vi "Close Private Data Cluster Refs.vi"(8 "error in (no error)":errorcluster, 11 "Private Data Refs":T1) -> (0 "error out":errorcluster)   [LabVIEW 2020, in "Add to Private Data.lvlib"]
uses:
  Add to Private Data.lvlib
  Private Data Refs.ctl
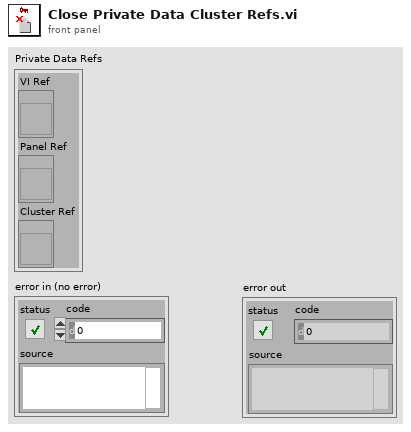
[diagram p1: front panel]
types:
  T1 = typedef "Add to Private Data.lvlib/Private Data Refs.ctl" = cluster{"VI Ref":refnum<vi>, "Panel Ref":refnum<vi>, "Cluster Ref":refnum<vi>}
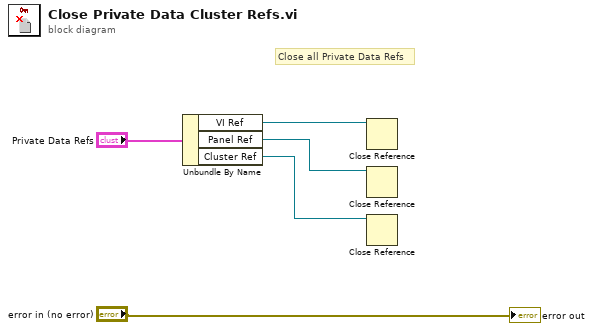
[diagram p0: block diagram]
diagram:
  # "Close all Private Data Refs"
  n1 = Unbundle By Name("Private Data Refs") -> ("VI Ref"=w3:refnum<vi>, "Panel Ref"=w2:refnum<vi>, "Cluster Ref"=w1:refnum<vi>)
  n2 = Close Reference(reference=w3) -> ()  [unwired: 1 in, 1 out]
  n3 = Close Reference(reference=w2) -> ()  [unwired: 1 in, 1 out]
  n4 = Close Reference(reference=w1) -> ()  [unwired: 1 in, 1 out]
  "error out" <- "error in (no error)"
